vi "Camera Acquisition Listner FG.vi"(8 "error in":errorcluster, 11 "Camera Selector":T2=enum."Bottom") -> (0 "error out":errorcluster, 3 "Acq Loop Listner":T1=enum."User Interface")   [LabVIEW 2012]
doc: "Returns an image space for a given camera index."
uses:
  MsgQ Loops enum.ctl
  Main MsgQ.lvlib
  Image Acquisition/CAMERA NAME ENUM.ctl
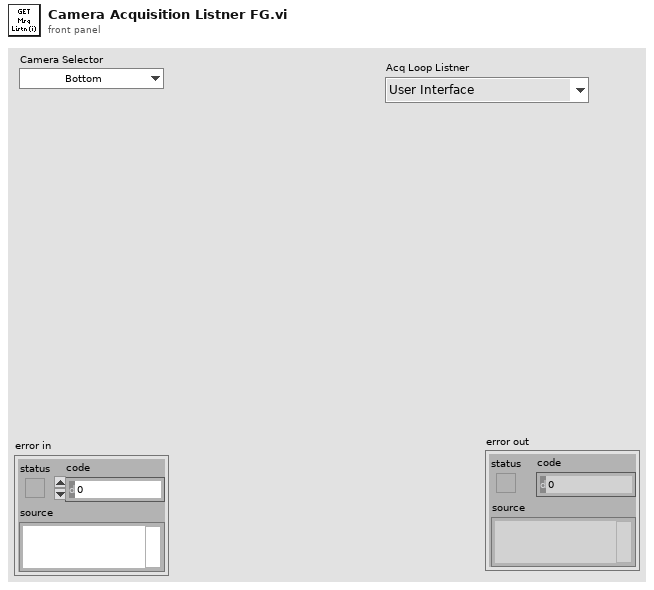
[diagram p1: front panel]
types:
  T1 = typedef "Main MsgQ.lvlib/MsgQ Loops enum.ctl" = enum16{"I2C", "TCP", "User Interface", "File IO", "Pattern Sequence", "Oscope"}
  T2 = typedef "CAMERA NAME ENUM.ctl" = enum16{"Top", "Bottom", "Left", "Right"}
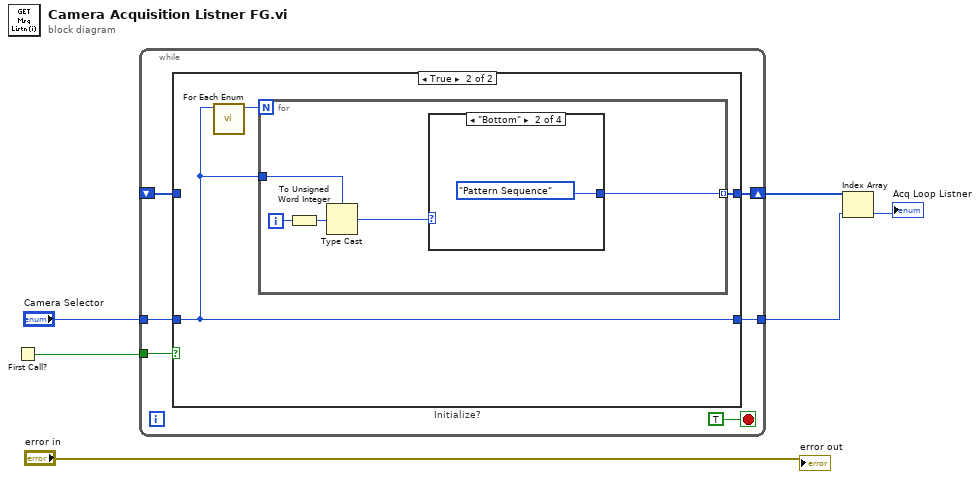
[diagram p0: block diagram]
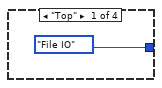
[diagram p3: hidden frame]
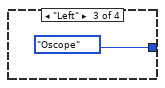
[diagram p4: hidden frame]
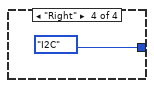
[diagram p5: hidden frame]
diagram:
  n1 = First Call?() -> (First Call?: T/F=w5:bool)
  n2 = while {
    tunnel: w5 -> [w11]
    shift-right: [w10] -> w4
    shift-left: _ -> [w9]
    tunnel: "Camera Selector" -> [w8]
    tunnel: [w7] -> w2
    stop <- TRUE stop-if-true
    n3 = case "Initialize?" shown="True" w11 {
      tunnel: [w14 w15] -> w10
      tunnel: w9 -> [w14 _]
      tunnel: w8 -> [w13 w16]
      tunnel: [w13 w16] -> w7
      frame False {
      }
      frame True {
        n4 = call "For Each Enum.vi"("Enum In"=w16) -> ("# elements"=w17:i32)  [unwired: 9 in, 1 out]
        n5 = for {
          N: w17 -> [_]
          tunnel: w16 -> [w20]
          tunnel: [w18] -> w15 mode=indexing
          i -> [w22]
          n6 = To Unsigned Word Integer(number=w22) -> (unsigned 16bit integer=w21:u16)
          n7 = Type Cast(type=w20, x=w21) -> (*(type *) &x=w19:T2)
          n8 = case shown="\"Bottom\"" w19 {
            tunnel: [MsgQ_Loops_enum."File IO" ("Send to MsgQ") MsgQ_Loops_enum."Pattern Sequence" ("Send to MsgQ") MsgQ_Loops_enum."Oscope" ("Send to MsgQ") MsgQ_Loops_enum."I2C" ("Send to MsgQ")] -> w18
            frame "Top" {
            }
            frame "Bottom" {
            }
            frame "Left" {
            }
            frame "Right" {
            }
          }
        }
      }
    }
  }
  n9 = Index Array(array=w4, index=w2) -> (element=→"Acq Loop Listner":T1)
  "error out" <- "error in"
